vi "Part 2.vi"(11 "Input":string) -> (3 "Output":i64)   [LabVIEW 2021]
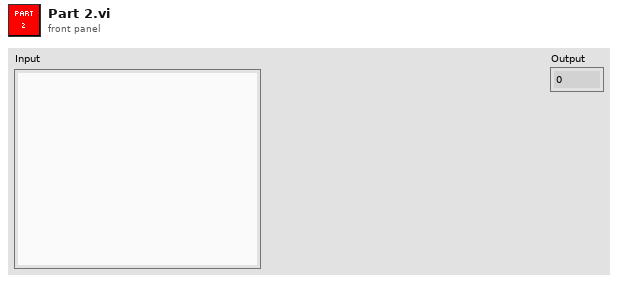
[diagram p1: front panel]
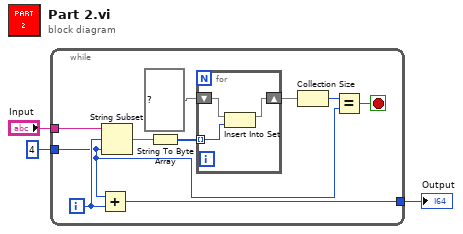
[diagram p0: block diagram]
diagram:
  n1 = while {
    tunnel: "Input" -> [w13]
    tunnel: 4 ("length (rest)") -> [w5]
    tunnel: [w4] -> w1
    i -> [w6]
    stop <- w7 stop-if-true
    n2 = Add(x=w5, y=w6) -> (x+y=w4:i32)
    n3 = String Subset(string=w13, offset (0)=w6, length (rest)=w5) -> (substring=w12:string)
    n4 = String To Byte Array(string=w12) -> (unsigned byte array=w11:u8[])
    n5 = for {
      tunnel: w11 -> [w16] mode=indexing
      shift-right: [w14] -> w9
      shift-left: set{u8} {} ("set in") -> [w15]
      n6 = Insert Into Set(10:w16, 11:w15) -> (3:w14:set{u8})  [unwired: 1 out]
    }
    n7 = Collection Size(1:w9) -> (0:w8:i32)
    n8 = Equal?(x=w8, y=w5) -> (x = y?=w7:bool)
  }
  "Output" <- w1
